vi "SemiGreedy_Filters_(Top_Level_VI)-6.vi"(5 "[IN] Max angle":dbl, 6 "[IN] Dot matrix with statuses \nfor potentially moving dots":i16[][](array[numeric]), 7 "[IN] Possibly\nMoving (X,Y)":dbl[][](array[numeric]), 8 "error IN":errorcluster, 9 "[IN] Areas particles\nPrimary Detected":dbl[][](array[numeric]), 10 "[IN] Primary \n(X,Y) Detected":dbl[][](array[numeric]), 11 "[IN] Grouped tracks":T1(array[cluster])) -> (0 "error OUT":errorcluster, 2 "[OUT] Processed Tracks":T1(array[cluster]), 3 "[OUT Tracks before Processing":T1(array[cluster]))   [LabVIEW 2013]
panel:
  out "Numeric":i32
  out "# Iteration":i32
  out "Current\ngroup":i32
  out "# of corrections":i32
  out "[IN] Before Pro\ncessing Tracks":T1(array[cluster])
  out "[IN] Current Pro\ncessing Tracks":T2
  out "[OUT] Clusters for Re\nconstructed Tracks":T2
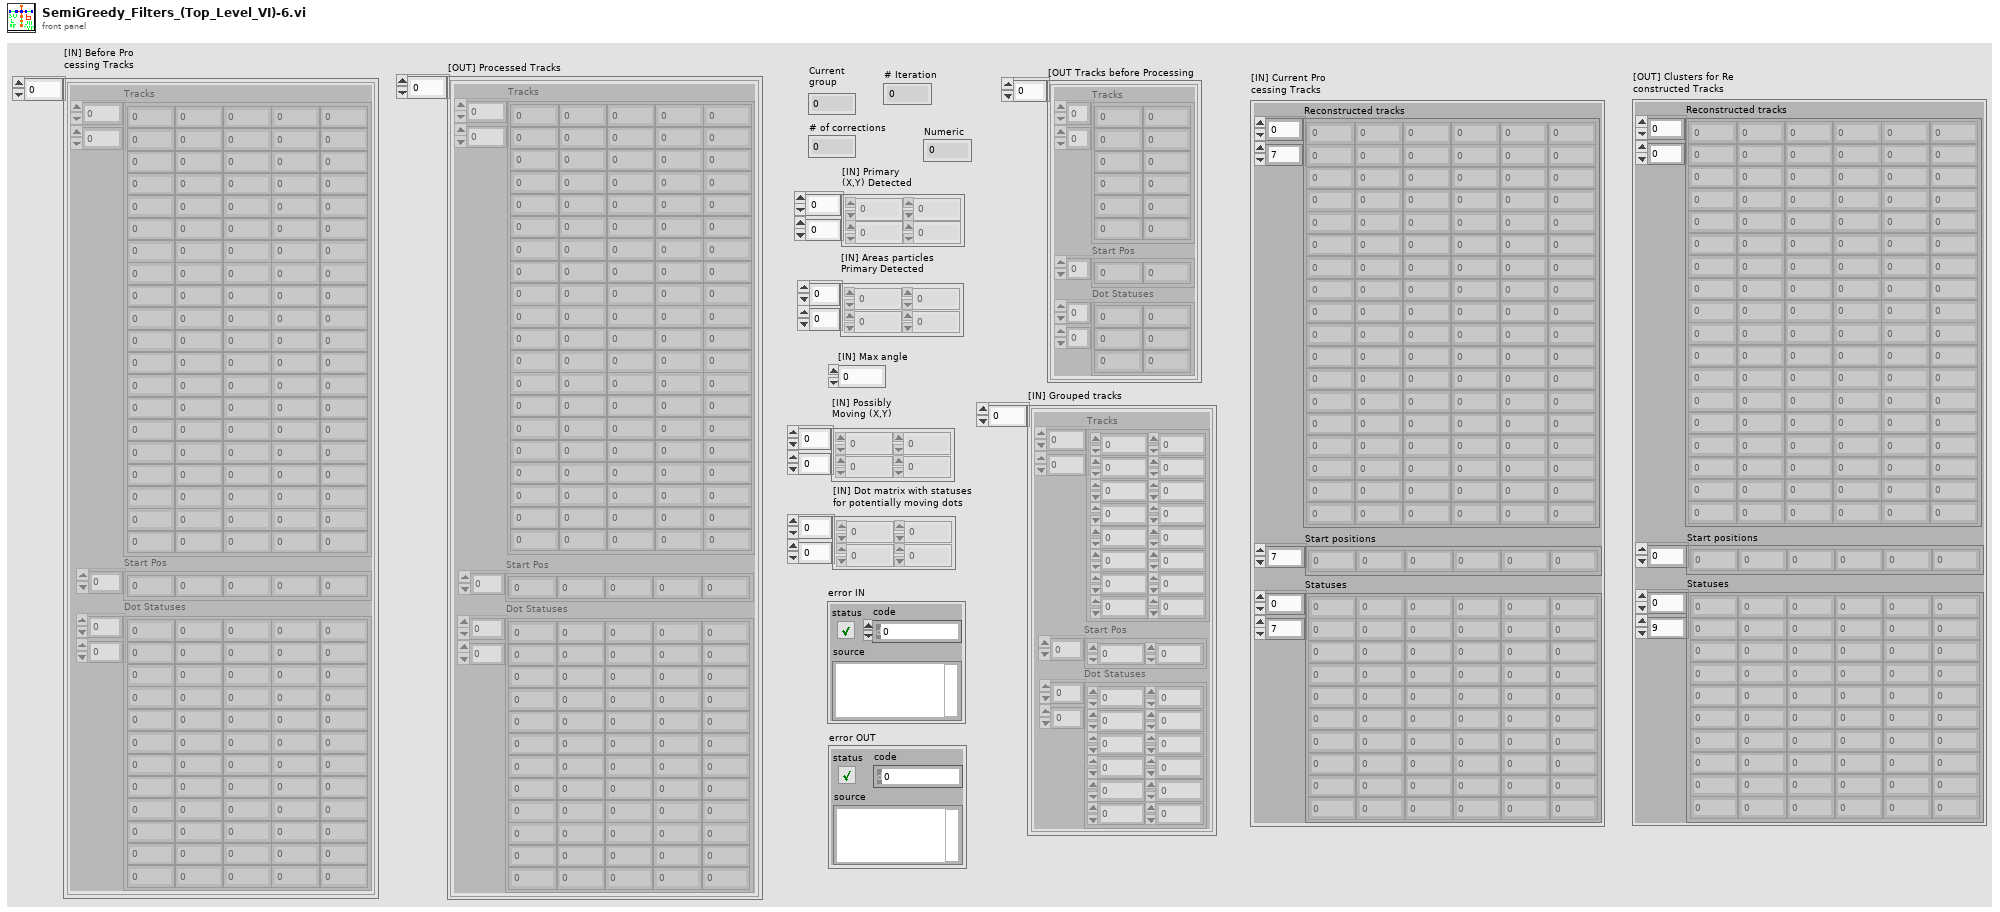
[diagram p1: front panel]
types:
  T1 = cluster{"Tracks":dbl[][], "Start Pos":i32[], "Dot Statuses":i16[][]}[]
  T2 = cluster{"Reconstructed tracks":dbl[][], "Start positions":i32[], "Statuses":i16[][]}
  T3 = cluster{"[IN] Possibly\nMoving (X,Y)":dbl[][], "[IN] Dot matrix with statuses \nfor potentially moving dots":i16[][], "[IN] Primary \n(X,Y) Detected ":dbl[][], "[IN] Max angle":dbl, "[IN] Areas particles\nPrimary Detected ":dbl[][]}
  T4 = cluster{"Tracks":dbl[][], "Start Pos":i32[], "Dot Statuses":i16[][]}
  T5 = cluster{"Subtrack":dbl[], "Statuses":i16[], "Start pos":i32, "Additions to cost":i8, "Track variant \nis too short":bool, "Indicies for Jumps":i32[]}[][]
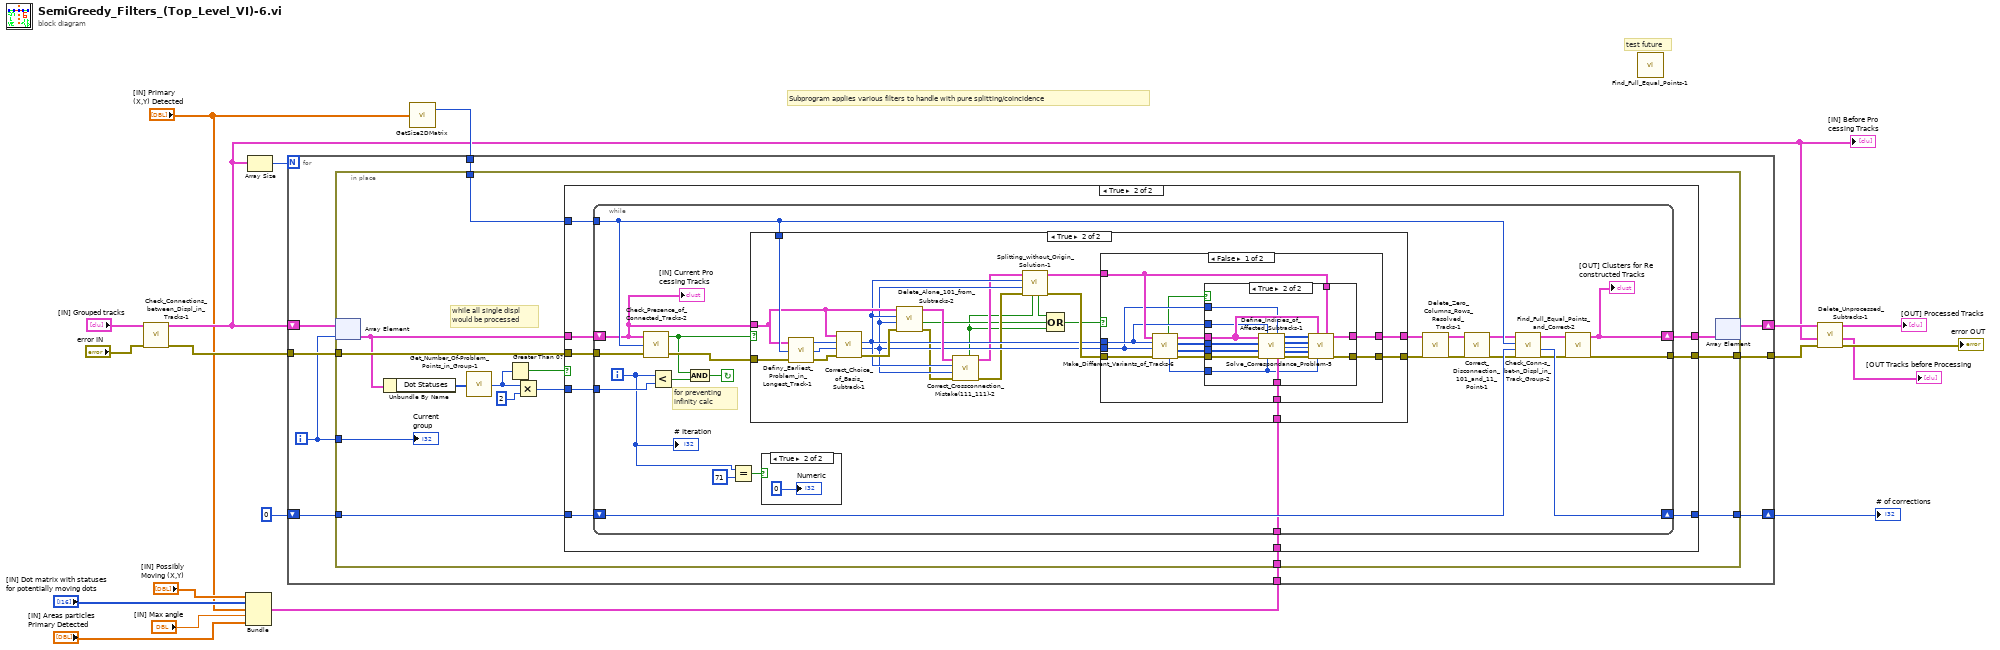
[diagram p0: block diagram]
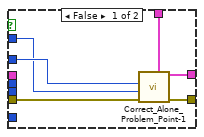
[diagram p5: hidden frame]
diagram:
  # "test future"
  # "Subprogram applies various filters to handle with pure splitting/coincidence"
  n1 = call "Check_Connections_between_Displ_in_Tracks-1.vi"("error IN"="error IN", "[IN] Long Connected Tracks"="[IN] Grouped tracks") -> ("error OUT"=w11:errorcluster, "[OUT] Long Connected Tracks"=w10:T1)  [unwired: 4 in]
  "[IN] Before Pro\ncessing Tracks" <- w10
  n2 = Bundle("[IN] Possibly\nMoving (X,Y)"="[IN] Possibly\nMoving (X,Y)", "[IN] Dot matrix with statuses \nfor potentially moving dots"="[IN] Dot matrix with statuses \nfor potentially moving dots", "[IN] Primary \n(X,Y) Detected"="[IN] Primary \n(X,Y) Detected", "[IN] Max angle"="[IN] Max angle", "[IN] Areas particles\nPrimary Detected"="[IN] Areas particles\nPrimary Detected") -> (w1:T3)  [unwired: 1 in]
  n3 = Array Size(array=w10) -> (size(s)=w19:i32)
  n4 = call "GetSize2DMatrix.vi"("Array IN (2D)"="[IN] Primary \n(X,Y) Detected") -> ("# Cols"=w16:i32)  [unwired: 1 out]
  n5 = for {
    N: w19 -> [_]
    shift-right: [w20] -> w15
    shift-left: w10 -> [w22]
    tunnel: w11 -> [w28]
    tunnel: w16 -> [w27]
    tunnel: [w26] -> w14
    shift-right: [w24] -> w7
    shift-left: 0 -> [w25]
    tunnel: w1 -> [w23]
    i -> [w21]
    n6 = in-place {
      in-place-border: w28 -> [w42]
      in-place-border: w27 -> [w41]
      in-place-border: [w40] -> w26
      in-place-border: w25 -> [w39]
      in-place-border: [w38] -> w24
      in-place-border: w23 -> [w35]
      in-place-border: w21 -> [w31]
      # "while all single displ\nwould be processed"
      n7 = in-place-array #1(w22, w21) -> (w30:T4)
      n8 = Unbundle By Name(w30) -> ("Dot Statuses"=w37:i16[][])
      n9 = call "Get_Number_Of-Problem_Points_in_Group-1.vi"("[IN] Dot Statuses"=w37) -> ("[OUT] Number of problem points"=w34:i32)
      n10 = Greater Than 0?(x=w34) -> (x > 0?=w36:bool)
      n11 = Multiply(x=w34, y=2) -> (x*y=w32:i32)
      n12 = case shown="True" w36 {
        tunnel: w42 -> [w44 w54]
        tunnel: w41 -> [_ w53]
        tunnel: [w44 w52] -> w40
        tunnel: [w45 w51] -> w29
        tunnel: w39 -> [w43 w50]
        tunnel: [w43 w49] -> w38
        tunnel: w30 -> [w45 w48]
        tunnel: w32 -> [_ w47]
        tunnel: w35 -> [_ w46]
        frame False {
        }
        frame True {
          n13 = while {
            tunnel: w54 -> [w71]
            tunnel: w53 -> [w68]
            shift-right: [w65] -> w51
            shift-left: w48 -> [w64]
            tunnel: [w67] -> w52
            shift-right: [w75] -> w49
            shift-left: w50 -> [w76]
            tunnel: w47 -> [w73]
            tunnel: w46 -> [w66]
            i -> [w55]
            stop <- w74 continue-if-true
            # "for preventing \ninfinity calc"
            n14 = call "Check_Presence_of_Connected_Tracks-2.vi"("error IN"=w71, "[IN] #of Frames"=w68, "[IN] Still connected\ntracks in group"=w64) -> ("error OUT"=w70:errorcluster, "[OUT] At least two tracks\ninside track group"=w69:bool)  [unwired: 1 in]
            n15 = Less?(x=w55, y=w73) -> (x < y?=w72:bool)
            n16 = And(x=w69, y=w72) -> (x .and. y?=w74:bool)
            n17 = Equal?(x=w55, y=71) -> (x = y?=w56:bool)
            n18 = case shown="True" w69 {
              tunnel: w70 -> [w80 w103]
              tunnel: w64 -> [w81 w96]
              tunnel: w68 -> [_ w102]
              tunnel: [w81 w101] -> w77
              tunnel: [w80 w100] -> w78
              tunnel: w66 -> [_ w94]
              frame False {
              }
              frame True {
                n19 = call "Definy_Earliest_Problem_in_Longest_Track-1.vi"("error IN"=w103, "[IN] #of Frames"=w102, "[IN] Still connected\ntracks in group"=w96) -> ("error OUT"=w97:errorcluster, "[OUT] # of Longest track\nInside the Group of Tracks"=w98:i32, "[OUT] Index of Problem\nPoint Inside Track"=w99:i32)
                n20 = call "Correct_Choice_of_Basis_Subtrack-1.vi"("error IN"=w97, "[IN] # of Longest track\nInside the Group of Tracks"=w98, "[IN] Index of Earliest \nProblem Point Inside"=w99, "[IN] Still connected\ntracks in group"=w96) -> ("error OUT"=w95:errorcluster, "[OUT] # of Correc\nted Longest Track"=w89:i32, "[OUT] # of Prob\nlem Point Inside"=w90:i32)  [unwired: 1 in]
                n21 = call "Delete_Alone_101_from_Subtracks-2.vi"("error IN"=w95, "[IN] # of Correc\nted Longest Track"=w89, "[IN] # of Prob\nlem Point Inside"=w90, "[IN] Still connected\ntracks in group"=w96) -> ("error OUT"=w88:errorcluster, "[OUT] Special case: \nAlone 101 point"=w83:bool, "[OUT] Clusters for Re\nconstructed Tracks"=w91:T2)  [unwired: 1 in]
                n22 = call "Correct_Crossconnection_Mistake(111_111)-2.vi"("error IN"=w88, "[IN] # of Track with\nFirst Problem Point"=w89, "[IN] Index of First Pro\nblem Point Inside Track"=w90, "[IN] Still connected\ntracks in group"=w91) -> ("error OUT"=w87:errorcluster, "[OUT] Clusters for Re\nconstructed Tracks"=w86:T2, "[OUT] Crossconn\nection corrected"=w82:bool)  [unwired: 5 in]
                n23 = call "Splitting_without_Origin_Solution-1.vi"("[IN] Crossconn\nection corrected"=w82, "error IN"=w87, "[IN] # of Track with\nFirst Problem Point"=w89, "[IN] Index of First Pro\nblem Point Inside Track"=w90, "[IN] Still connected\ntracks in group"=w86) -> ("error OUT"=w92:errorcluster, "[OUT] Clusters for Re\nconstructed Tracks"=w93:T2, "[OUT] Problem with 11 Point\nwithout Origin Resolved"=w85:bool)  [unwired: 4 in]
                n24 = Compound Arithmetic op=OR(w85, w83, w82) -> (w84:bool)
                n25 = case shown="False" w84 {
                  tunnel: [w106 w140] -> w101
                  tunnel: [w105 w139] -> w100
                  tunnel: w90 -> [w108 _]
                  tunnel: w89 -> [w107 _]
                  tunnel: w92 -> [w116 w139]
                  tunnel: w93 -> [w110 w140]
                  tunnel: w94 -> [w115 _]
                  frame False {
                    n26 = call "Make_Different_Variants_of_Tracks-6.vi"("error IN"=w116, "[IN] # of Longest track\nInside the Group of Tracks"=w107, "[IN] Index of Earliest \nProblem Point Inside"=w108, "[IN] Still connected\ntracks in group"=w110) -> ("error OUT"=w114:errorcluster, "[OUT] Index of # tracks \nwith problem points"=w113:i32[], "[OUT] Index of connected \npoints inside the track"=w109:i32[], "[OUT] Subtracks"=w111:T5, "[OUT] Status of 1st Problem Point"=w112:i16, "[OUT] 2 or more subtracks"=w104:bool)  [unwired: 2 in]
                    n27 = case shown="True" w104 {
                      tunnel: w115 -> [_ w138]
                      tunnel: w114 -> [w119 w137]
                      tunnel: w113 -> [_ w136]
                      tunnel: w112 -> [_ w134]
                      tunnel: w111 -> [_ w131]
                      tunnel: w110 -> [w122 w130]
                      tunnel: w109 -> [_ w129]
                      tunnel: w108 -> [w118 w128]
                      tunnel: w107 -> [w117 w127]
                      tunnel: [w121 w124] -> w106
                      tunnel: [w120 w123] -> w105
                      frame False {
                        n28 = call "Correct_Alone_Problem_Point-1.vi"("[IN] # of Prob\nlem Point Inside"=w118, "[IN] # of Longest track\nInside the Group of Tracks"=w117, "error IN"=w119, "[IN] Still connected\ntracks in group"=w122) -> ("[OUT] Clusters for Re\nconstructed Tracks"=w121:T2, "error OUT"=w120:errorcluster)  [unwired: 3 in]
                      }
                      frame True {
                        n29 = call "Define_Indicies_of_Affected_Subtracks-1.vi"("[IN] Subtracks"=w131, "[IN] # of Prob\nlem Point Inside"=w128, "[IN] # of Longest track\nInside the Group of Tracks"=w127, "[IN] Index of connected \npoints inside the track"=w129, "[IN] Index of # tracks \nwith problem points"=w136, "error IN"=w137, "[IN] Status of 1st Problem Point"=w134, "[IN] Values for Cost F() Calc"=w138) -> ("[OUT] Indicies of \nPoints Inside Trks"=w125:i32[], "[OUT] Indicies of \nall Affected Tracks\n(initial point =0)"=w126:i32[], "[OUT] Index of Optimal \nSubtrack Splitting Case"=w133:i32, "[OUT] Optimal solution \nfor Merging Case"=w132:i32[], "error OUT"=w135:errorcluster)  [unwired: 3 in]
                        n30 = call "Solve_Correspondance_Problem-5.vi"("[IN] Indicies of Po\nints Inside Trks"=w125, "[IN] Subtracks"=w131, "[IN] Still connected\ntracks in group"=w130, "[IN] Indicies of all \nAffected Tracks \n(initial point = 0)"=w126, "[IN] Index of Optimal \nSubtrack Splitting Case"=w133, "[IN] Optimal solution \nfor Merging Case"=w132, "error IN"=w135, "[IN] Status of 1st \nProblem Point"=w134) -> ("[OUT] Clusters for Re\nconstructed Tracks"=w124:T2, "error OUT"=w123:errorcluster)  [unwired: 6 in]
                      }
                    }
                  }
                  frame True {
                  }
                }
              }
            }
            n31 = case shown="True" w56 {
              frame False {
              }
              frame True {
                "Numeric" <- 0
              }
            }
            n32 = call "Delete_Zero_Columns_Rows_Resolved_Tracks-1.vi"("error IN"=w78, "[IN] Clusters for Re\nconstructed Tracks"=w77) -> ("error OUT"=w60:errorcluster, "[OUT] Clusters for Re\nconstructed Tracks"=w61:T2)  [unwired: 4 in]
            n33 = call "Correct_Disconnection_101_and_11_Point-1.vi"("error IN"=w60, "[IN] Still connected\ntracks in group"=w61) -> ("error OUT"=w58:errorcluster, "[OUT] Clusters for Re\nconstructed Tracks"=w59:T2)  [unwired: 4 in]
            n34 = call "Check_Conn-s_bet-n_Displ_in_Track_Group-2.vi"("error IN"=w58, "[IN] # of Unconne\ncted Problem points"=w76, "[IN] #of Frames"=w68, "[IN] Clusters for Re\nconstructed Tracks"=w59) -> ("error OUT"=w62:errorcluster, "[OUT] # of Unconne\ncted Problem points"=w75:i32, "[OUT] Clusters for Re\nconstructed Tracks"=w63:T2)  [unwired: 1 in]
            n35 = call "Find_Full_Equal_Points_and_Correct-2.vi"("error IN"=w62, "[IN] Clusters for Re\nconstructed Tracks"=w63) -> ("error OUT"=w67:errorcluster, "[OUT] Clusters for Re\nconstructed Tracks"=w65:T2)  [unwired: 4 in]
            "[OUT] Clusters for Re\nconstructed Tracks" <- w65
            "# Iteration" <- w55
            "[IN] Current Pro\ncessing Tracks" <- w64
          }
        }
      }
      n36 = in-place-array #1(w29) -> (w20:T1)  [unwired: 1 out]
      "Current\ngroup" <- w31
    }
  }
  "# of corrections" <- w7
  n37 = call "Find_Full_Equal_Points-1.vi"() -> ()  [unwired: 6 in, 2 out]
  n38 = call "Delete_Unprocessed_Subtracks-1.vi"("error IN"=w14, "[IN] Before Pro\ncessing Tracks"=w10, "[IN] Processed Tracks"=w15) -> ("error OUT"=→"error OUT":errorcluster, "[OUT] Before Pro\ncessing Tracks"=→"[OUT Tracks before Processing":T1, "[IN] Filtered Tracks"=→"[OUT] Processed Tracks":T1)  [unwired: 2 in]
